vi "Find First Matching Resource (String).vi"(6 "Error if not found? (F)":bool, 8 "error in (no error)":errorcluster, 10 "Resource Types":string[](array[string]), 11 "Resources":T1[](array[typedef])) -> (0 "error out":errorcluster, 1 "Index":i32, 2 "Resource":T1, 3 "Resources out":T1[](array[typedef]), 5 "Found?":bool)   [LabVIEW 2026, in "VILab.lvlib"]
uses:
  VILab.lvlib
  CTLs/Resource.ctl
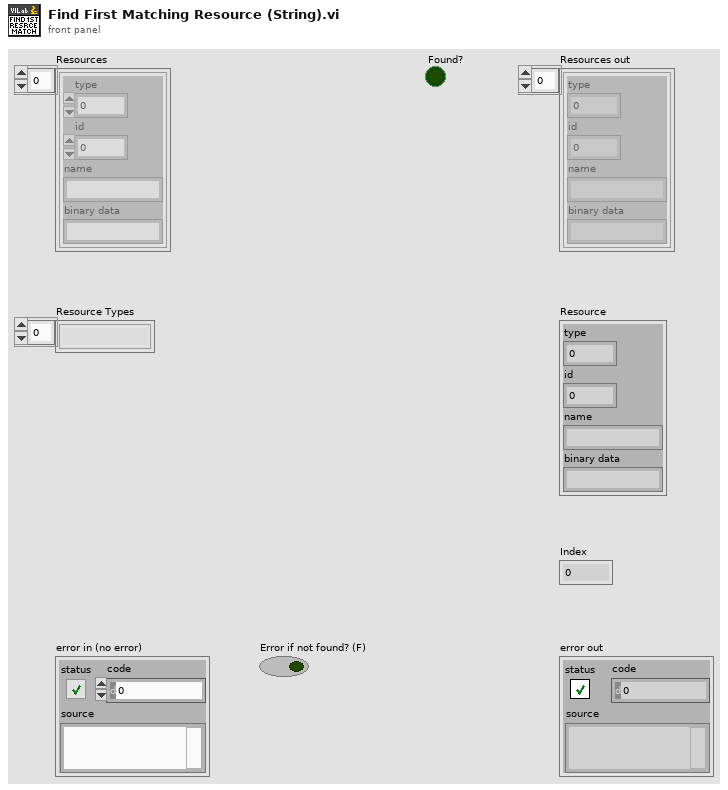
[diagram p1: front panel]
types:
  T1 = typedef "VILab.lvlib/Resource.ctl" = cluster{"type":u32, "id":i32, "name":string, "binary data":string}
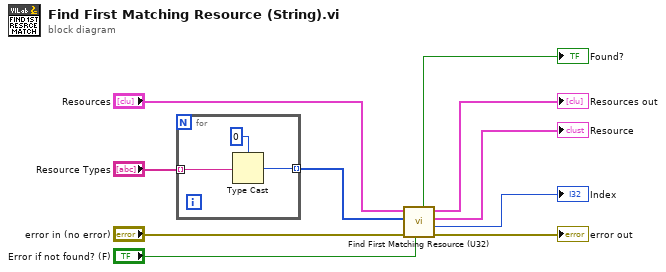
[diagram p0: block diagram]
diagram:
  n1 = for {
    tunnel: "Resource Types" -> [w12] mode=indexing
    tunnel: [w11] -> w8 mode=indexing
    n2 = Type Cast(type=u32 0, x=w12) -> (*(type *) &x=w11:u32)
  }
  n3 = call "Find First Matching Resource (U32).vi"("Error if not found? (F)"="Error if not found? (F)", "error in (no error)"="error in (no error)", "Resource Types"=w8, "Resources"="Resources") -> ("error out"=→"error out":errorcluster, "Index"=→"Index":i32, "Resource"=→"Resource":T1, "Resources out"=→"Resources out":T1[], "Found?"=→"Found?":bool)  [unwired: 3 in]
